vi "http 414 Request URI Too Long.vi"(11 "application request in":T3) -> (3 "application request out":T1)   [LabVIEW 2016, in "Basic HTTPS server.lvclass"]
uses:
  Basic HTTPS server.lvclass
  http response.ctl
  http response packet type.ctl
  HTTP headers/http header data.ctl
  HTTP headers/http headers.lvlib
  http method.ctl
  http request.ctl
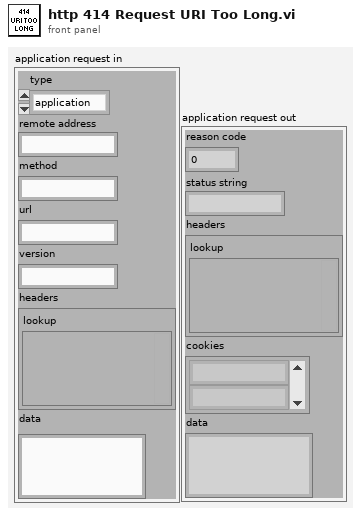
[diagram p1: front panel]
types:
  T1 = typedef "Basic HTTPS server.lvclass/http response.ctl" = cluster{"reason code":u16, "status string":string, "headers":T2, "cookies":string[], "data":string}
  T2 = typedef "http headers.lvlib/http header data.ctl" = cluster{"lookup":variant}
  T3 = typedef "Basic HTTPS server.lvclass/http request.ctl" = cluster{"type":T4, "remote address":string, "method":string, "url":string, "version":string, "headers":T2, "data":string}
  T4 = typedef "Basic HTTPS server.lvclass/http method.ctl" = enum16{"application", "error", "upgrade"}
  T5 = typedef "Basic HTTPS server.lvclass/http response packet type.ctl" = enum16{"full response", "header only", "data only", "last data", "raw output"}
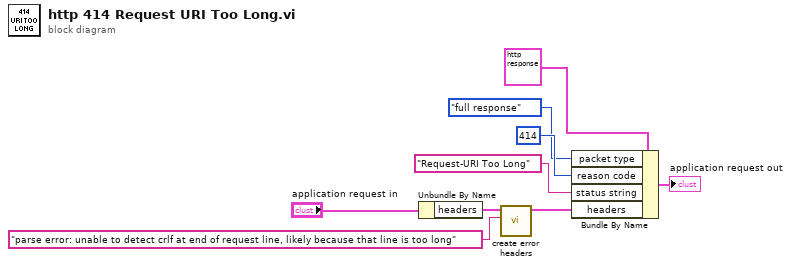
[diagram p0: block diagram]
diagram:
  n1 = Unbundle By Name("application request in") -> ("headers"=w1:T2)
  n2 = call "create error headers.vi"("custom error reason"="parse error: unable to detect crlf at end of request line, likely because that line is too long" ("name"), "headers in"=w1) -> ("headers out"=w4:T2)  [unwired: 9 in]
  n3 = Bundle By Name(cluster=T1 {"reason code"=0, "status string"="", "headers"={"lookup"=variant}, "cookies"=[], "data"=""} ("application request"), "packet type"=http_response_packet_type."full response", "reason code"=u16 414, "status string"="Request-URI Too Long", "headers"=w4) -> (→"application request out":T1)
